vi "CameraGuidage[withfinetune](V4.56).vi"(0 "NumX in":i16=657, 1 "StartX":i16=1, 3 "Mode":u16(ring) items=["Exposition Guideur"=0, "Guidage"=2, "Piedestal"=3, "Exposition simple"=4, "Stop Guidage"=5, "Calibration"=8], 4 "Duration":dbl=0.40000000000000013 min=0.0 step=0.1 format="%.2f", 5 "BinX":i16=1, 6 "NumberofImg":i32=1 caption="Nombre d'image" min=1 step=1, 7 "MaxIm.ICCDCamera":refnum<k7>, 9 "BinY":i16=1, 11 "NumY in":i16=495, 12 "StartY":i16=1, 14 "GuiderDeclination":i16) -> (8 "Done":bool, 10 "Error":errorcluster, 15 "GuiderArrayError":errorcluster)   [LabVIEW 2011]
uses:
  Globals.vi
panel:
  out "GuiderUpdate":bool=TRUE
  out "SaveImage":bool
  out "DarkImg":i32[][](array[numeric])
  in  "removedark":bool
  out "NumY dark":i16=495
  out "NumX dark":i16=657
  out "NumY out":i16=495
  out "NumX out":i16=657
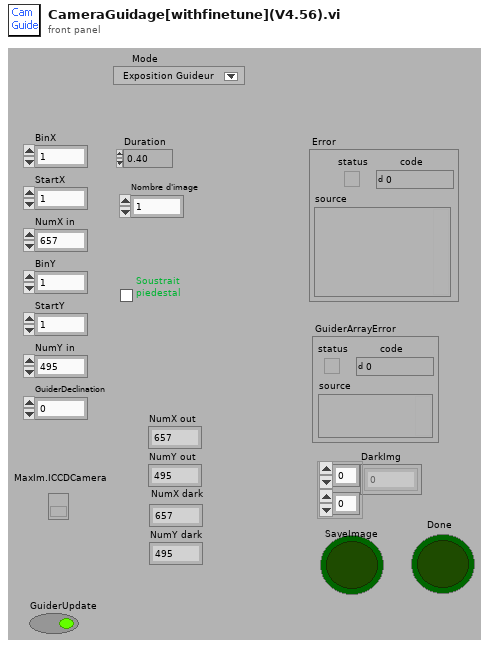
[diagram p1: front panel]
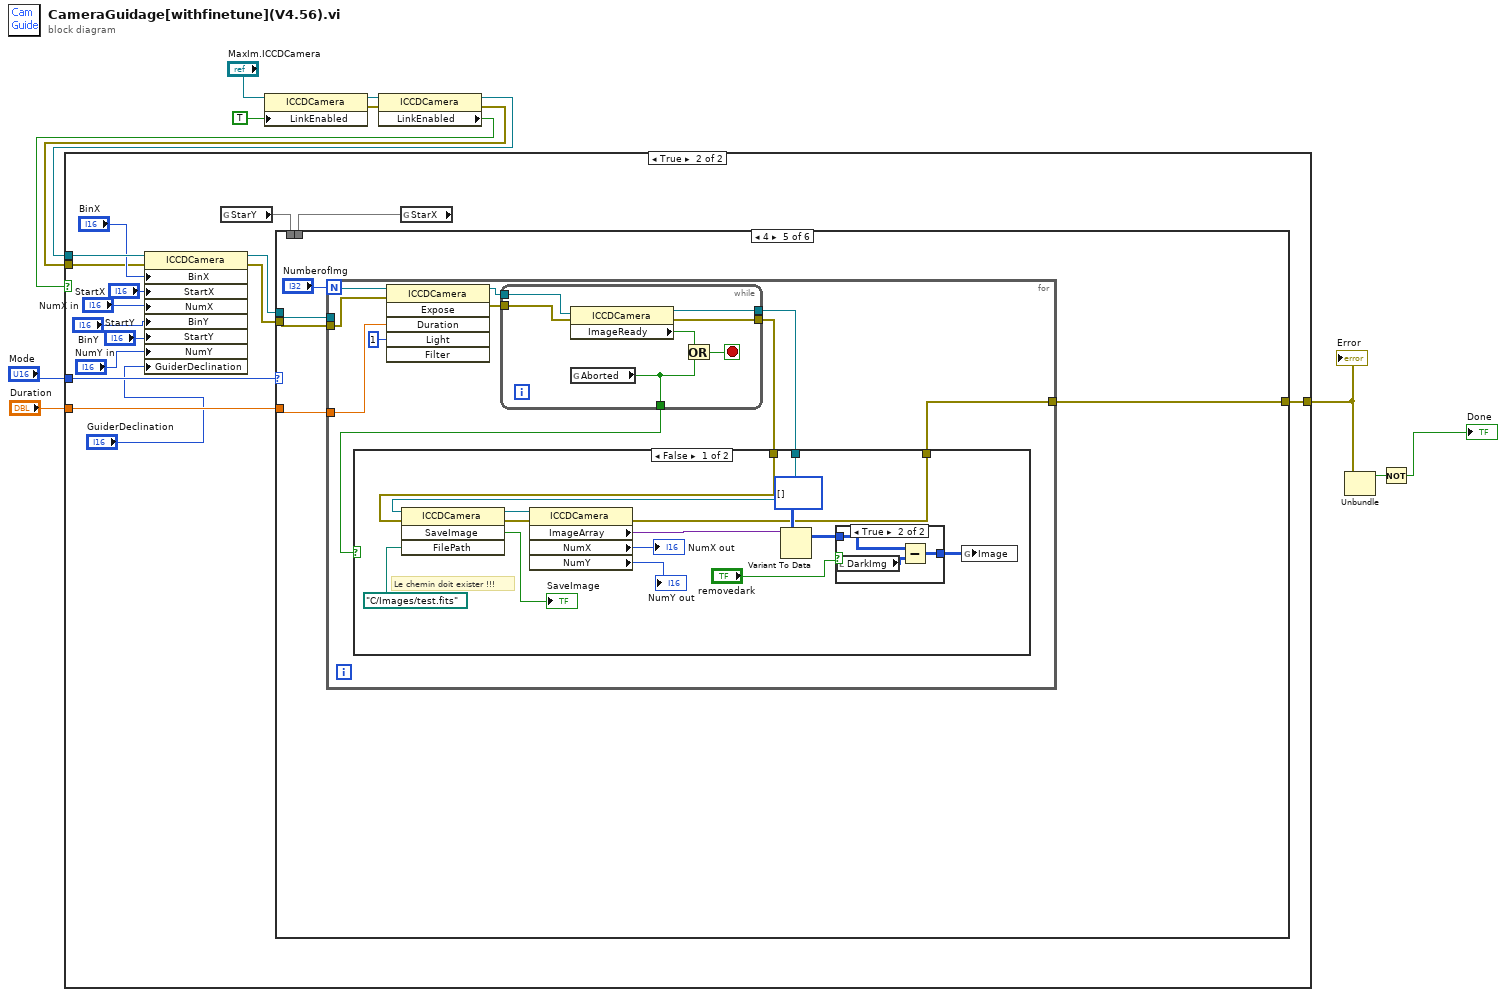
[diagram p0: block diagram]
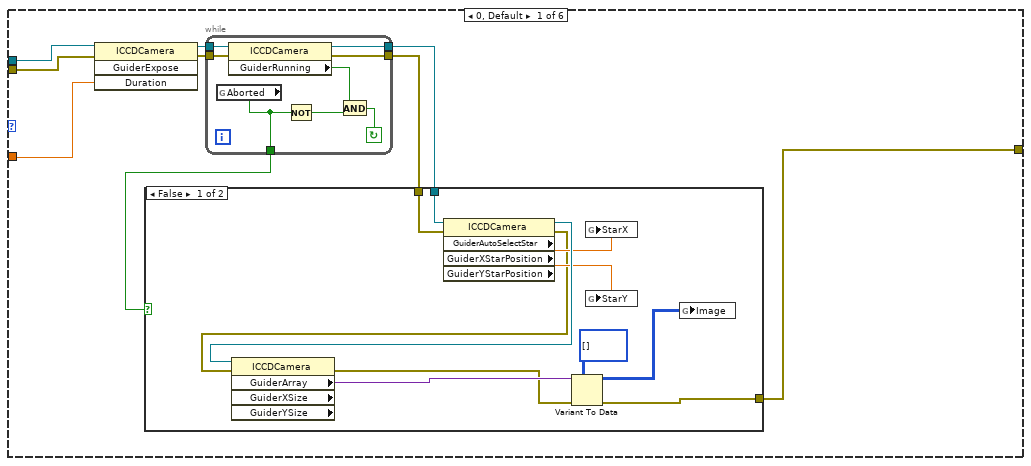
[diagram p3: hidden frame]
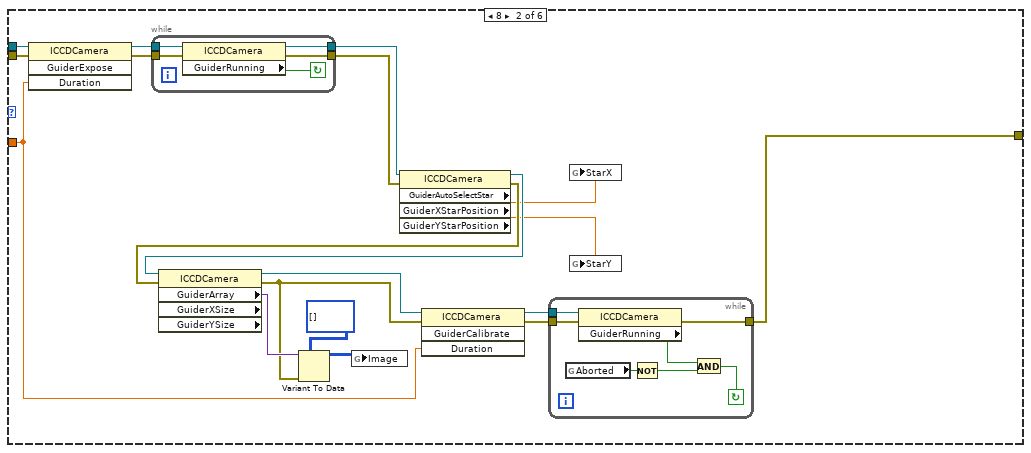
[diagram p5: hidden frame]
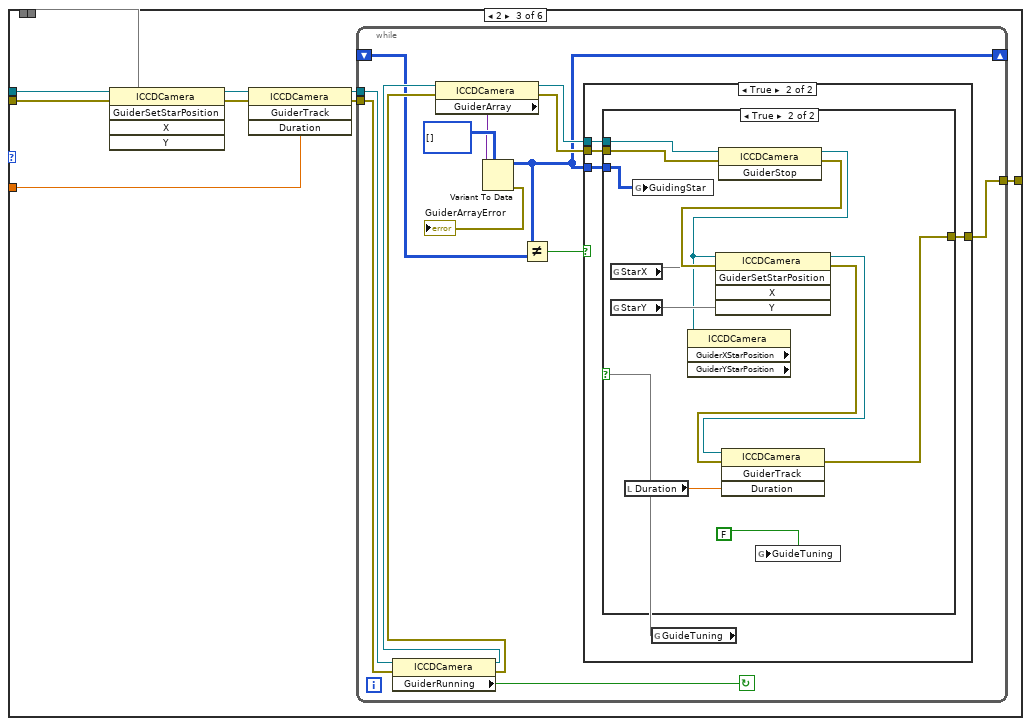
[diagram p6: hidden frame]
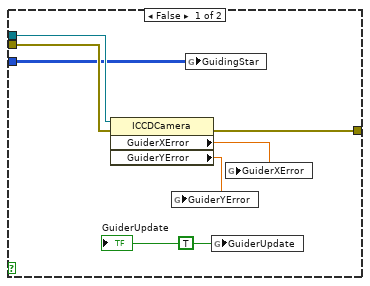
[diagram p8: hidden frame]
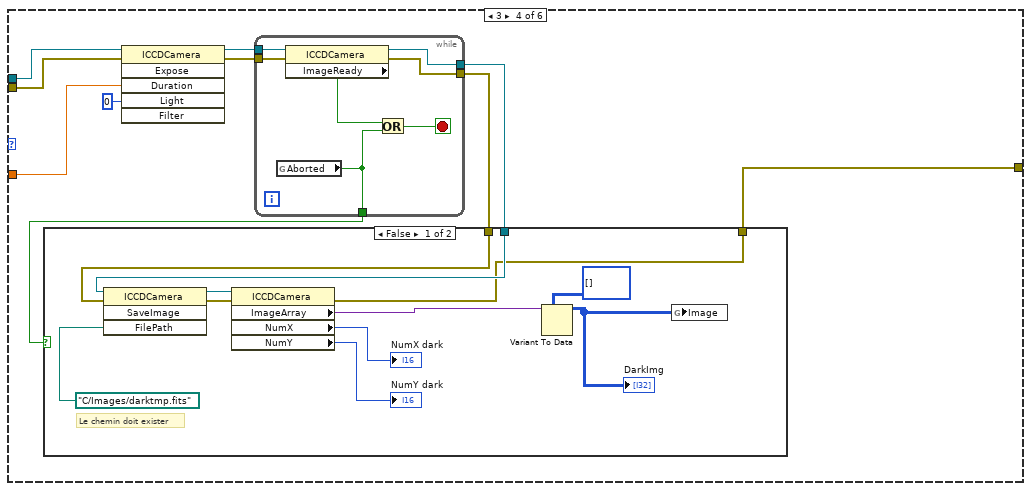
[diagram p9: hidden frame]
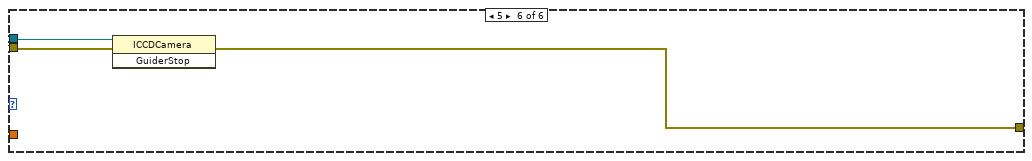
[diagram p13: hidden frame]
diagram:
  n1 = property class="ICCDCamera"(reference="MaxIm.ICCDCamera", "LinkEnabled"=TRUE) -> (reference out=w5:refnum<k7>, error out=w1:errorcluster)  [unwired: 1 in]
  n2 = property class="ICCDCamera"(reference=w5, error in=w1) -> (reference out=w10:refnum<k7>, error out=w9:errorcluster, "LinkEnabled"=w8:bool)
  n3 = case shown="True" w8 {
    tunnel: w10 -> [_ w27]
    tunnel: "Duration" -> [_ w29]
    tunnel: w9 -> [w13 w15]
    tunnel: [w13 w14] -> w6
    tunnel: "Mode" -> [_ w28]
    frame False {
    }
    frame True {
      n4 = property class="ICCDCamera"(reference=w27, error in=w15, "BinX"="BinX", "StartX"="StartX", "NumX"="NumX in", "BinY"="BinY", "StartY"="StartY", "NumY"="NumY in", "GuiderDeclination"="GuiderDeclination") -> (reference out=w26:refnum<k7>, error out=w25:errorcluster)
      n5 = global read "Globals.vi" "StarY"() -> (w16)
      n6 = global read "Globals.vi" "StarX"() -> (w17)
      n7 = case shown="4" w28 {
        tunnel: w26 -> [w35 w66 w94 w146 w172 w211]
        tunnel: w29 -> [w36 w62 w99 w143 w171 _]
        tunnel: w25 -> [w34 w65 w93 w142 w170 w210]
        tunnel: [w30 w75 w96 w140 w168 w209] -> w14
        tunnel: w17 -> [_ _ w91 _ _ _]
        tunnel: w16 -> [_ _ w90 _ _ _]
        frame 0, Default {
          n8 = invoke class="ICCDCamera" method="GuiderExpose"(reference=w35, error in=w34, "Duration"=w36) -> (reference out=w38:refnum<k7>, error out=w32:errorcluster)  [unwired: 1 in, 2 out]
          n9 = while {
            tunnel: [w55] -> w31
            tunnel: w32 -> [w56]
            tunnel: [w57] -> w37
            tunnel: w38 -> [w58]
            tunnel: [w51] -> w33
            stop <- w54 continue-if-true
            n10 = global read "Globals.vi" "Aborted"() -> (w51:bool)
            n11 = property class="ICCDCamera"(reference=w58, error in=w56) -> (reference out=w57:refnum<k7>, error out=w55:errorcluster, "GuiderRunning"=w53:bool)
            n12 = Not(x=w51) -> (.not. x?=w52:bool)
            n13 = And(x=w53, y=w52) -> (x .and. y?=w54:bool)
          }
          n14 = case shown="False" w33 {
            tunnel: w37 -> [w49 _]
            tunnel: w31 -> [w48 w50]
            tunnel: [w40 w50] -> w30
            frame False {
              n15 = property class="ICCDCamera" props=["GuiderAutoSelectStar", "GuiderXStarPosition", "GuiderYStarPosition"](reference=w49, error in=w48) -> (reference out=w47:refnum<k7>, error out=w39:errorcluster, "GuiderXStarPosition"=w43:sgl, "GuiderYStarPosition"=w42:sgl)  [unwired: 1 out]
              n16 = property class="ICCDCamera" props=["GuiderArray", "GuiderXSize", "GuiderYSize"](reference=w47, error in=w39) -> (error out=w41:errorcluster, "GuiderArray"=w46:variant)  [unwired: 3 out]
              n17 = Variant To Data(error in=w41, type=i32[][] [], Variant=w46) -> (data=w44:i32[][], error out=w40:errorcluster)
              n18 = global write "Globals.vi" "StarX"(w43) -> ()
              n19 = global write "Globals.vi" "StarY"(w42) -> ()
              n20 = global write "Globals.vi" "Image"(w44) -> ()
            }
            frame True {
            }
          }
        }
        frame 8 {
          n21 = invoke class="ICCDCamera" method="GuiderExpose"(reference=w66, error in=w65, "Duration"=w62) -> (reference out=w74:refnum<k7>, error out=w73:errorcluster)  [unwired: 1 in, 2 out]
          n22 = while {
            tunnel: [w79] -> w71
            tunnel: w73 -> [w80]
            tunnel: [w81] -> w72
            tunnel: w74 -> [w82]
            stop <- w78 continue-if-true
            n23 = property class="ICCDCamera"(reference=w82, error in=w80) -> (reference out=w81:refnum<k7>, error out=w79:errorcluster, "GuiderRunning"=w78:bool)
          }
          n24 = property class="ICCDCamera" props=["GuiderAutoSelectStar", "GuiderXStarPosition", "GuiderYStarPosition"](reference=w72, error in=w71) -> (reference out=w70:refnum<k7>, error out=w69:errorcluster, "GuiderXStarPosition"=w59:sgl, "GuiderYStarPosition"=w60:sgl)  [unwired: 1 out]
          n25 = property class="ICCDCamera" props=["GuiderArray", "GuiderXSize", "GuiderYSize"](reference=w70, error in=w69) -> (reference out=w64:refnum<k7>, error out=w63:errorcluster, "GuiderArray"=w68:variant)  [unwired: 2 out]
          n26 = Variant To Data(error in=w63, type=u32[][] [], Variant=w68) -> (data=w61:u32[][])  [unwired: 1 out]
          n27 = global write "Globals.vi" "Image"(w61) -> ()
          n28 = invoke class="ICCDCamera" method="GuiderCalibrate"(reference=w64, error in=w63, "Duration"=w62) -> (reference out=w77:refnum<k7>, error out=w76:errorcluster)  [unwired: 1 in, 2 out]
          n29 = while {
            tunnel: [w87] -> w75
            tunnel: w76 -> [w88]
            tunnel: w77 -> [w89]
            stop <- w83 continue-if-true
            n30 = global read "Globals.vi" "Aborted"() -> (w86:bool)
            n31 = property class="ICCDCamera"(reference=w89, error in=w88) -> (error out=w87:errorcluster, "GuiderRunning"=w85:bool)  [unwired: 1 out]
            n32 = Not(x=w86) -> (.not. x?=w84:bool)
            n33 = And(x=w85, y=w84) -> (x .and. y?=w83:bool)
          }
          n34 = global write "Globals.vi" "StarX"(w59) -> ()
          n35 = global write "Globals.vi" "StarY"(w60) -> ()
        }
        frame 2 {
          n36 = invoke class="ICCDCamera" method="GuiderSetStarPosition"(reference=w94, error in=w93, "X"=w91, "Y"=w90) -> (reference out=w95:refnum<k7>, error out=w92:errorcluster)  [unwired: 1 in, 3 out]
          n37 = invoke class="ICCDCamera" method="GuiderTrack"(reference=w95, error in=w92, "Duration"=w99) -> (reference out=w98:refnum<k7>, error out=w97:errorcluster)  [unwired: 1 in, 2 out]
          n38 = while {
            tunnel: [w111] -> w96
            tunnel: w97 -> [w112]
            tunnel: w98 -> [w113]
            shift-right: [w100] -> _
            shift-left: _ -> [w102]
            stop <- w110 continue-if-true
            n39 = property class="ICCDCamera"(reference=w113, error in=w112) -> (reference out=w107:refnum<k7>, error out=w106:errorcluster, "GuiderRunning"=w110:bool)
            n40 = property class="ICCDCamera"(reference=w107, error in=w106) -> (reference out=w108:refnum<k7>, error out=w109:errorcluster, "GuiderArray"=w103:variant)
            n41 = Variant To Data(type=i16[][] [], Variant=w103) -> (data=w100:i16[][], error out=→"GuiderArrayError":errorcluster)  [unwired: 1 in]
            n42 = Not Equal?(x=w100, y=w102) -> (x != y?=w104:bool)
            n43 = case shown="True" w104 {
              tunnel: w109 -> [w114 w117]
              tunnel: w108 -> [_ w118]
              tunnel: [w114 w119] -> w111
              tunnel: w100 -> [_ w116]
              frame False {
              }
              frame True {
                n44 = global read "Globals.vi" "GuideTuning"() -> (w115)
                n45 = case shown="True" w115 {
                  tunnel: [w126 w135] -> w119
                  tunnel: w118 -> [w122 w138]
                  tunnel: w117 -> [w121 w137]
                  tunnel: w116 -> [w120 w133]
                  frame False {
                    w123 = TRUE ("GuiderUpdate")
                    n46 = property class="ICCDCamera"(reference=w122, error in=w121) -> (error out=w126:errorcluster, "GuiderXError"=w125:sgl, "GuiderYError"=w124:sgl)  [unwired: 1 out]
                    n47 = global write "Globals.vi" "GuiderYError"(w124) -> ()
                    n48 = global write "Globals.vi" "GuidingStar"(w120) -> ()
                    n49 = global write "Globals.vi" "GuiderUpdate"(w123) -> ()
                    n50 = global write "Globals.vi" "GuiderXError"(w125) -> ()
                    "GuiderUpdate" <- w123
                  }
                  frame True {
                    n51 = global read "Globals.vi" "StarX"() -> (w129)
                    n52 = global read "Globals.vi" "StarY"() -> (w128)
                    n53 = local read "Duration"() -> (w136:dbl)
                    n54 = global write "Globals.vi" "GuidingStar"(w133) -> ()
                    n55 = invoke class="ICCDCamera" method="GuiderStop"(reference=w138, error in=w137) -> (reference out=w127:refnum<k7>, error out=w132:errorcluster)  [unwired: 1 in, 1 out]
                    n56 = property class="ICCDCamera" props=["GuiderXStarPosition", "GuiderYStarPosition"](reference=w127) -> ()  [unwired: 1 in, 4 out]
                    n57 = invoke class="ICCDCamera" method="GuiderSetStarPosition"(reference=w127, error in=w132, "X"=w129, "Y"=w128) -> (reference out=w131:refnum<k7>, error out=w130:errorcluster)  [unwired: 1 in, 3 out]
                    n58 = invoke class="ICCDCamera" method="GuiderTrack"(reference=w131, error in=w130, "Duration"=w136) -> (error out=w135:errorcluster)  [unwired: 1 in, 3 out]
                    n59 = global write "Globals.vi" "GuideTuning"(FALSE) -> ()
                  }
                }
              }
            }
          }
        }
        frame 3 {
          n60 = invoke class="ICCDCamera" method="Expose"(reference=w146, error in=w142, "Duration"=w143, "Light"=i16 0) -> (reference out=w148:refnum<k7>, error out=w145:errorcluster)  [unwired: 2 in, 4 out]
          n61 = while {
            tunnel: [w164] -> w144
            tunnel: w145 -> [w165]
            tunnel: [w166] -> w147
            tunnel: w148 -> [w167]
            tunnel: [w161] -> w139
            stop <- w163 stop-if-true
            n62 = global read "Globals.vi" "Aborted"() -> (w161:bool)
            n63 = property class="ICCDCamera"(reference=w167, error in=w165) -> (reference out=w166:refnum<k7>, error out=w164:errorcluster, "ImageReady"=w162:bool)
            n64 = Or(x=w162, y=w161) -> (x .or. y?=w163:bool)
          }
          n65 = case shown="False" w139 {
            tunnel: w147 -> [w159 _]
            tunnel: w144 -> [w158 w160]
            tunnel: [w151 w160] -> w140
            frame False {
              # "Le chemin doit exister"
              n66 = invoke class="ICCDCamera" method="SaveImage"(reference=w159, error in=w158, "FilePath"=path "C:/Images/darktmp.fits") -> (reference out=w157:refnum<k7>, error out=w154:errorcluster)  [unwired: 1 in, 2 out]
              n67 = property class="ICCDCamera"(reference=w157, error in=w154) -> (error out=w151:errorcluster, "ImageArray"=w156:variant, "NumX"=→"NumX dark":i16, "NumY"=→"NumY dark":i16)  [unwired: 1 out]
              n68 = Variant To Data(type=i32[][] [], Variant=w156) -> (data=w149:i32[][])  [unwired: 1 in, 1 out]
              "DarkImg" <- w149
              n69 = global write "Globals.vi" "Image"(w149) -> ()
            }
            frame True {
            }
          }
        }
        frame 4 {
          n70 = for {
            N: "NumberofImg" -> [_]
            tunnel: w172 -> [w180]
            tunnel: w171 -> [w177]
            tunnel: [w176] -> w168
            tunnel: w170 -> [w175]
            n71 = invoke class="ICCDCamera" method="Expose"(reference=w180, error in=w175, "Duration"=w177, "Light"=i16 1) -> (reference out=w182:refnum<k7>, error out=w179:errorcluster)  [unwired: 2 in, 4 out]
            n72 = while {
              tunnel: [w205] -> w178
              tunnel: w179 -> [w206]
              tunnel: [w207] -> w181
              tunnel: w182 -> [w208]
              tunnel: [w202] -> w173
              stop <- w204 stop-if-true
              n73 = property class="ICCDCamera"(reference=w208, error in=w206) -> (reference out=w207:refnum<k7>, error out=w205:errorcluster, "ImageReady"=w203:bool)
              n74 = global read "Globals.vi" "Aborted"() -> (w202:bool)
              n75 = Or(x=w203, y=w202) -> (x .or. y?=w204:bool)
            }
            n76 = case shown="False" w173 {
              tunnel: w181 -> [w196 _]
              tunnel: w178 -> [w195 w201]
              tunnel: [w188 w201] -> w176
              frame False {
                # "Le chemin doit exister !!!"
                n77 = invoke class="ICCDCamera" method="SaveImage"(reference=w196, error in=w195, "FilePath"=path "C:/Images/test.fits") -> (reference out=w194:refnum<k7>, error out=w189:errorcluster, "SaveImage"=→"SaveImage":bool)  [unwired: 1 in, 1 out]
                n78 = property class="ICCDCamera"(reference=w194, error in=w189) -> (error out=w188:errorcluster, "ImageArray"=w193:variant, "NumX"=→"NumX out":i16, "NumY"=→"NumY out":i16)  [unwired: 1 out]
                n79 = Variant To Data(type=i32[][] [], Variant=w193) -> (data=w185:i32[][])  [unwired: 1 in, 1 out]
                n80 = case shown="True" "removedark" {
                  tunnel: w185 -> [w197 w200]
                  tunnel: [w197 w198] -> w184
                  frame False {
                  }
                  frame True {
                    n81 = local read "DarkImg"() -> (w199:i32[][])
                    n82 = Subtract(x=w200, y=w199) -> (x-y=w198:i32[][])
                  }
                }
                n83 = global write "Globals.vi" "Image"(w184) -> ()
              }
              frame True {
              }
            }
          }
        }
        frame 5 {
          n84 = invoke class="ICCDCamera" method="GuiderStop"(reference=w211, error in=w210) -> (error out=w209:errorcluster)  [unwired: 1 in, 2 out]
        }
      }
    }
  }
  "Error" <- w6
  n85 = Unbundle(w6) -> ("status"=w4:bool)  [unwired: 2 out]
  n86 = Not(x=w4) -> (.not. x?=→"Done":bool)
